vi "DataTranslation_NM1.vi"() -> ()   [LabVIEW 2011]
doc: "This vi will take data with multiple DT boxes for an arbitrary number of channels either differentially or single ended, depending upon how you have wired the boxes up."
uses:
  Controls/DT_Cluster.ctl
  Controls/DT_Mode.ctl
  Controls/Trigger_Mode.ctl
  Globals/Meas_global.vi
  <userlib>/LV-Link3/PolySubVIs/DtOLTimingSetInput.vi
  <userlib>/LV-Link3/PolySubVIs/DtCreateAinChan.vi
  <userlib>/LV-Link3/PolySubVIs/DtCreateCtrRateChan.vi
  <userlib>/LV-Link3/PolySubVIs/DtOLStartNormal.vi
  <userlib>/LV-Link3/PolySubVIs/DtOLReadMultiple2D.vi
  <userlib>/LV-Link3/PolySubVIs/DtOLTriggerDigital.vi
panel:
  out "DAQ Error":errorcluster
  out "Array":T1[](array[typedef])
  out "Clock Task":i32
  out "Waveform Graph":dbl[][](graph)
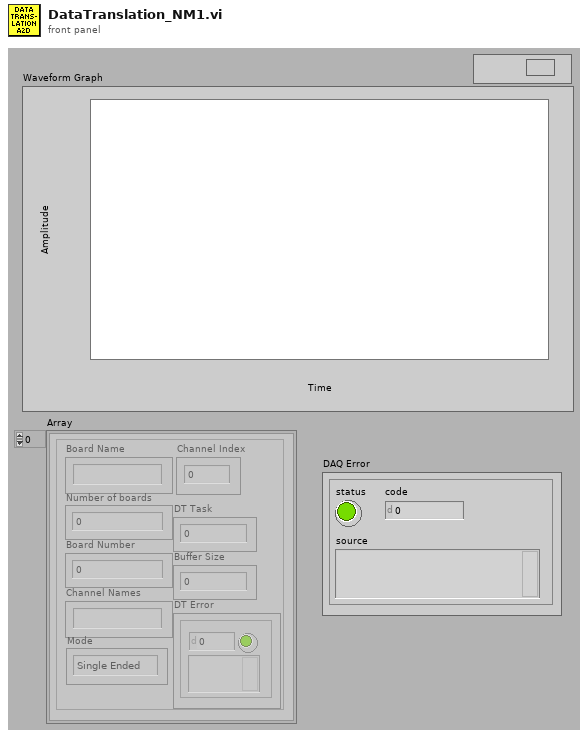
[diagram p1: front panel]
types:
  T1 = typedef "DT_Cluster.ctl" = cluster{"Board Name":string, "Number of boards":u32, "Board Number":u32, "Channel Names":string, "Channel Index":i32[], "DT Task":i32, "DT Error":errorcluster, "Mode":T2, "Buffer Size":u32}
  T2 = typedef "DT_Mode.ctl" = enum16{"Single Ended", "Differential"}
  T3 = typedef "Trigger_Mode.ctl" = enum16{"Free Running", "Start on Trigger", "Trigger Every Block", "Trigger Every Sample"}
  T4 = enum32{"Internal Clock", "External Clock", "No Timing"}
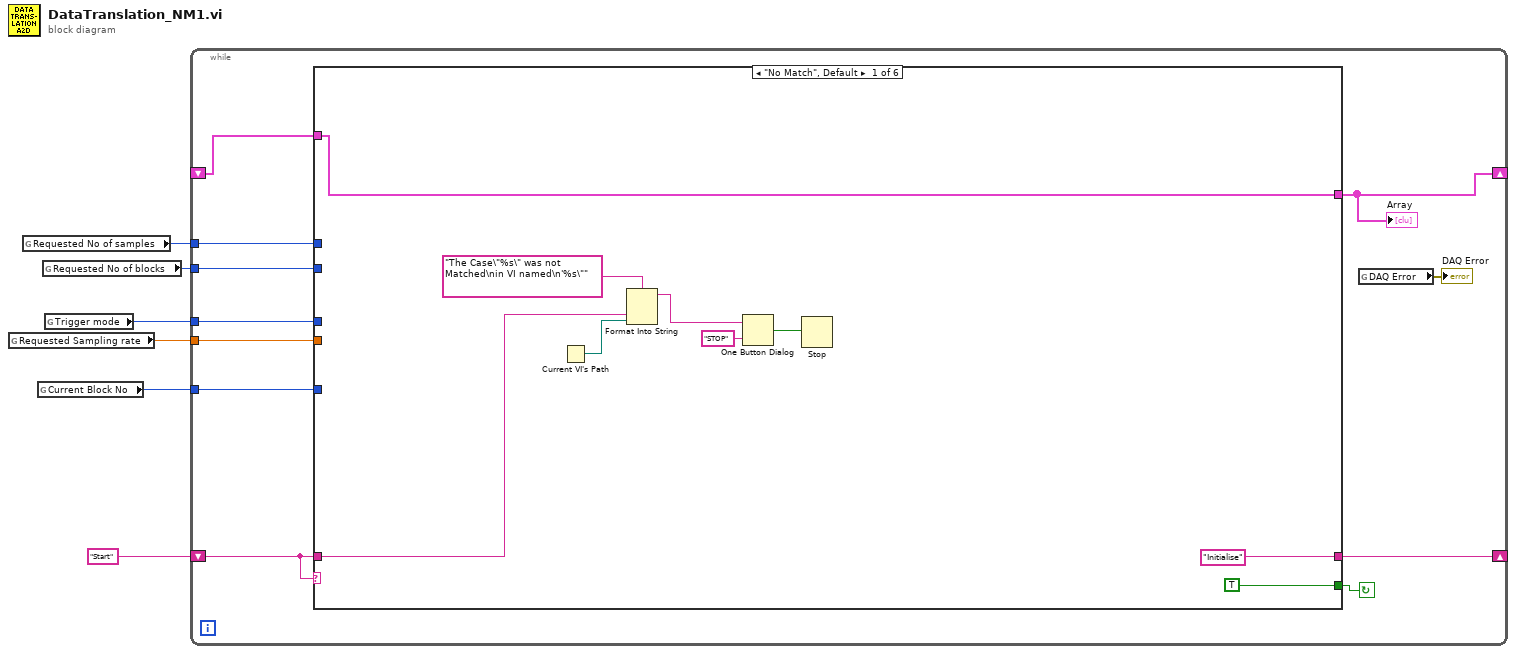
[diagram p0: block diagram]
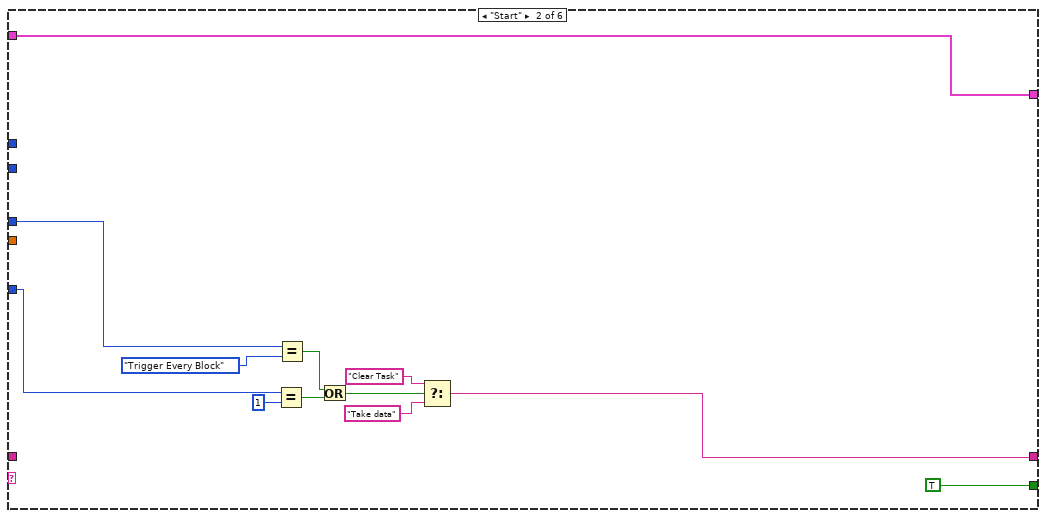
[diagram p2: hidden frame]
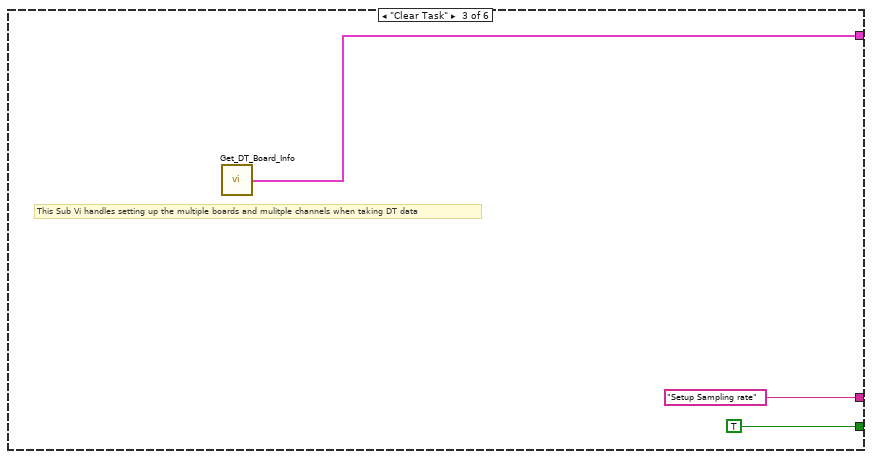
[diagram p3: hidden frame]
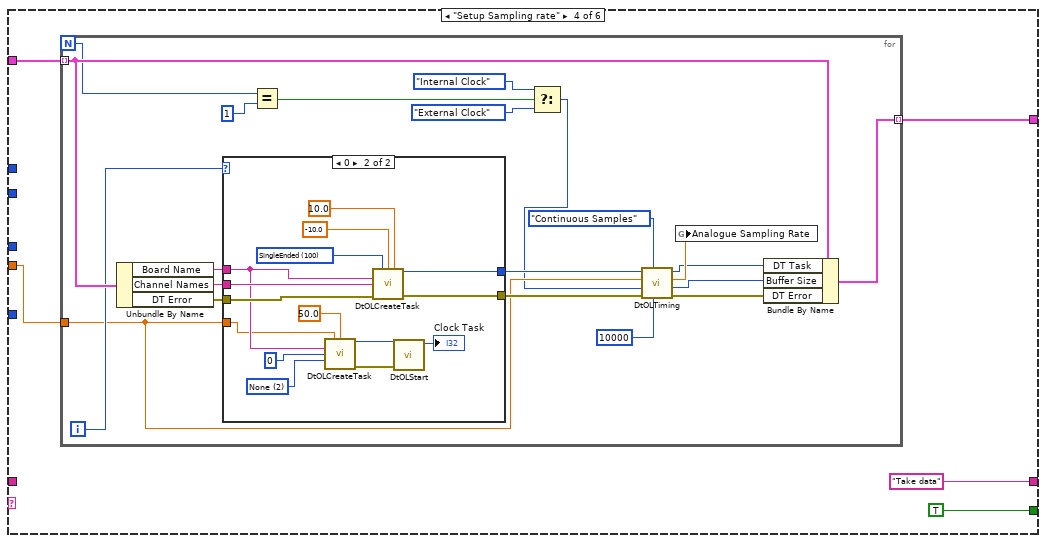
[diagram p4: hidden frame]
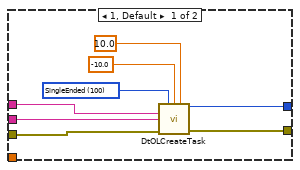
[diagram p5: hidden frame]
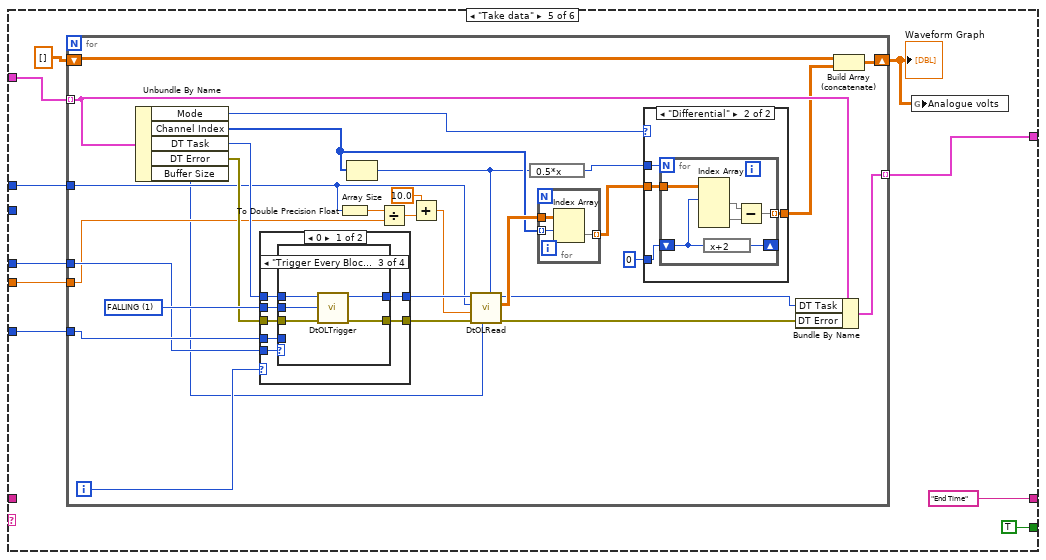
[diagram p6: hidden frame]
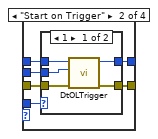
[diagram p9: hidden frame]
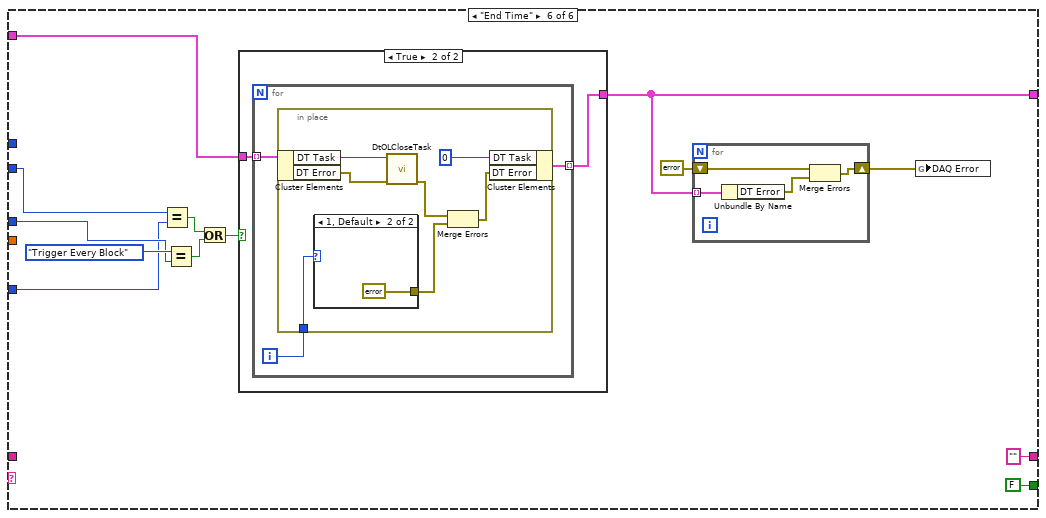
[diagram p13: hidden frame]
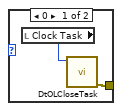
[diagram p15: hidden frame]
diagram:
  n1 = global read "Meas_global.vi" "Requested Sampling rate"() -> (w5:dbl)
  n2 = global read "Meas_global.vi" "Requested No of samples"() -> (w4:i32)
  n3 = global read "Meas_global.vi" "Current Block No"() -> (w2:i32)
  n4 = global read "Meas_global.vi" "Requested No of blocks"() -> (w1:i32)
  n5 = global read "Meas_global.vi" "Trigger mode"() -> (w3:T3)
  n6 = while {
    shift-left: "Start" -> [w16]
    shift-right: [w17] -> _
    tunnel: w5 -> [w15]
    tunnel: w4 -> [w14]
    tunnel: w2 -> [w13]
    tunnel: w3 -> [w11]
    tunnel: w1 -> [w10]
    shift-right: [w9] -> _
    shift-left: _ -> [w8]
    stop <- w12 continue-if-true
    n7 = case shown="\"No Match\", Default" w16 {
      tunnel: ["Initialise" w38 "Setup Sampling rate" "Take data" "End Time" "" ("f")] -> w17
      tunnel: w16 -> [w22 _ _ _ _ _]
      tunnel: w15 -> [_ _ _ w46 w92 _]
      tunnel: w14 -> [_ _ _ _ w99 _]
      tunnel: w13 -> [_ w34 _ _ w97 w180]
      tunnel: [TRUE TRUE TRUE TRUE TRUE FALSE] -> w12
      tunnel: w11 -> [_ w32 _ _ w96 w181]
      tunnel: w10 -> [_ _ _ _ _ w182]
      tunnel: w8 -> [w18 w27 _ w43 w95 w178]
      tunnel: [w18 w27 w39 w42 w94 w177] -> w9
      frame "No Match", Default {
        (unwired) FALSE
        n8 = Current VI's Path() -> (path=w21:path)
        n9 = Format Into String(format string="The Case\"%s\" was not Matched\nin VI named\n'%s\"" ("Format String"), w22, w21) -> (resulting string=w25:string)  [unwired: 2 in, 1 out]
        n10 = One Button Dialog(message=w25, button name ("OK")="STOP") -> (true=w23:bool)
        n11 = Stop(stop? (T)=w23) -> ()
      }
      frame "Start" {
        (unwired) TRUE
        n12 = Equal?(x=w34, y=1) -> (x = y?=w30:bool)
        n13 = Equal?(x=w32, y=Trigger_Mode."Trigger Every Block") -> (x = y?=w29:bool)
        n14 = Or(x=w29, y=w30) -> (x .or. y?=w28:bool)
        n15 = Select(t="Clear Task", s=w28, f="Take data") -> (s? t:f=w38:string)
      }
      frame "Clear Task" {
        (unwired) TRUE
        # "This Sub Vi handles setting up the multiple boards and mulitple channels when taking DT data"
        n16 = call "Get_DT_Board_Info.vi"() -> ("DT Cluster Array"=w39:T1[])  [unwired: 5 in]
      }
      frame "Setup Sampling rate" {
        n17 = for {
          N -> [w52]
          tunnel: w46 -> [w53]
          tunnel: w43 -> [w60] mode=indexing
          tunnel: [w59] -> w42 mode=indexing
          i -> [w54]
          n18 = Unbundle By Name(w60) -> ("Board Name"=w63:string, "Channel Names"=w62:string, "DT Error"=w61:errorcluster)
          n19 = case shown="0" w54 {
            tunnel: [w75 w90] -> w66
            tunnel: [w74 w89] -> w65
            tunnel: w63 -> [w73 w83]
            tunnel: w62 -> [w72 w88]
            tunnel: w61 -> [w71 w87]
            tunnel: w53 -> [_ w76]
            frame 1, Default {
              w68 = 100 items=["SingleEnded"=100, "Differential"=101] ("Channel Type")
              n20 = call-poly <userlib>:"DtOLCreateTask.vi"("Channel Type"=w68, "Range Min"=-10.0, "Range Max"=10.0, "Board Name"=w73, "Channel"=w72, "error in (no error)"=w71) -> ("Task out"=w74:i32, "error out"=w75:errorcluster)  [unwired: 7 in, 1 out]
            }
            frame 0 {
              w81 = 2 items=["LowLevel", "HighLevel", "None"] ("Gate Type")
              w84 = 100 items=["SingleEnded"=100, "Differential"=101] ("Channel Type")
              n21 = call-poly <userlib>:"DtOLCreateTask.vi"("Requested\nFrequency (Hz)"=w76, "Duty Cycle"=50.0, "Board Name"=w83, "Counter Num"=u32 0, "Gate Type"=w81) -> ("Task out"=w78:i32, "error out"=w79:errorcluster)  [unwired: 8 in, 1 out]
              n22 = call-poly <userlib>:"DtOLCreateTask.vi"("Channel Type"=w84, "Range Min"=-10.0, "Range Max"=10.0, "Board Name"=w83, "Channel"=w88, "error in (no error)"=w87) -> ("Task out"=w89:i32, "error out"=w90:errorcluster)  [unwired: 7 in, 1 out]
              n23 = call-poly <userlib>:"DtOLStart.vi"("error in (no error)"=w79, "Task in"=w78) -> ("Task out"=→"Clock Task":i32)  [unwired: 8 in, 1 out]
            }
          }
          n24 = Equal?(x=w52, y=1) -> (x = y?=w48:bool)
          n25 = Select(t=T4."Internal Clock" ("Timing"), s=w48, f=T4."External Clock" ("Timing")) -> (s? t:f=w47:T4)
          n26 = call-poly <userlib>:"DtOLTiming.vi"("Num Buffers"=u32 10000, "Sample Mode"=enum16{"Finite Samples", "Continuous Samples"}."Continuous Samples", "error in (no error)"=w66, "Timing"=w47, "Sample Freq (Hz)"=w53, "Task in"=w65) -> ("error out"=w55:errorcluster, "Buffer Size"=w56:u32, "Actual Sample Freq"=w58:dbl, "Task out"=w57:i32)  [unwired: 2 in]
          n27 = global write "Meas_global.vi" "Analogue Sampling Rate"(w58) -> ()
          n28 = Bundle By Name(cluster=w60, "DT Task"=w57, "Buffer Size"=w56, "DT Error"=w55) -> (w59:T1)
        }
      }
      frame "Take data" {
        n29 = for {
          tunnel: w99 -> [w112]
          tunnel: w97 -> [w127]
          tunnel: w96 -> [w126]
          tunnel: w95 -> [w122] mode=indexing
          tunnel: [w121] -> w94 mode=indexing
          shift-right: [w118] -> w91
          shift-left: dbl[][] [] -> [w117]
          tunnel: w92 -> [w113]
          i -> [w110]
          w128 = 1 items=["RISING", "FALLING"] ("External Trigger Polarity")
          n30 = Unbundle By Name(w122) -> ("Mode"=w106:T2, "Channel Index"=w119:i32[], "DT Task"=w125:i32, "DT Error"=w124:errorcluster, "Buffer Size"=w102:u32)
          n31 = case shown="0" w110 {
            tunnel: [w147 w171] -> w129
            tunnel: w128 -> [w146 _]
            tunnel: w127 -> [w145 _]
            tunnel: w126 -> [w144 _]
            tunnel: w125 -> [w143 w171]
            tunnel: w124 -> [w142 w170]
            tunnel: [w141 w170] -> w123
            frame 0 {
              n32 = case shown="\"Trigger Every Block\"" w144 {
                tunnel: [w149 w153 w165 w169] -> w147
                tunnel: w143 -> [w149 w154 w167 w169]
                tunnel: w145 -> [_ w155 _ _]
                tunnel: w146 -> [_ w152 w166 _]
                tunnel: w142 -> [w148 w151 w164 w168]
                tunnel: [w148 w150 w163 w168] -> w141
                frame "Free Running" {
                }
                frame "Start on Trigger" {
                  n33 = case shown="1" w155 {
                    tunnel: w154 -> [w160 w162]
                    tunnel: w151 -> [w159 w161]
                    tunnel: [w157 w162] -> w153
                    tunnel: [w158 w161] -> w150
                    tunnel: w152 -> [w156 _]
                    frame 1 {
                      n34 = call-poly <userlib>:"DtOLTrigger.vi"("error in (no error)"=w159, "External Trigger Polarity"=w156, "Task in"=w160) -> ("error out"=w158:errorcluster, "Task out"=w157:i32)  [unwired: 7 in]
                    }
                    frame 2, Default {
                    }
                  }
                }
                frame "Trigger Every Block" {
                  n35 = call-poly <userlib>:"DtOLTrigger.vi"("error in (no error)"=w164, "External Trigger Polarity"=w166, "Task in"=w167) -> ("error out"=w163:errorcluster, "Task out"=w165:i32)  [unwired: 7 in]
                }
                frame "Trigger Every Sample" {
                }
              }
            }
            frame 1, Default {
            }
          }
          n36 = To Double Precision Float(number=w112) -> (double precision float=w116:dbl)
          n37 = Array Size(array=w119) -> (size(s)=w104:i32)
          n38 = Divide(x=w116, y=w113) -> (x/y=w115:dbl)
          n39 = Add(x=10.0, y=w115) -> (x+y=w111:dbl)
          n40 = call-poly <userlib>:"DtOLRead.vi"("Number Chan to Read"=w104, "Buffer size"=w102, "error in (no error)"=w123, "Timeout"=w111, "Samples Per Channel"=w112, "Task in"=w129) -> ("error out"=w101:errorcluster, "2D Data out"=w120:dbl[][], "Task out"=w109:i32)  [unwired: 1 in, 2 out]
          n41 = expression code="0.5*x"(w104) -> (w103:i32)
          n42 = for {
            tunnel: w119 -> [w174] mode=indexing
            tunnel: w120 -> [w173]
            tunnel: [w172] -> w108 mode=indexing
            n43 = Index Array(array=w173, index (row)=w174) -> (element=w172:dbl[])  [unwired: 1 in]
          }
          n44 = case shown="\"Differential\"" w106 {
            tunnel: w108 -> [w130 w134]
            tunnel: [w130 w133] -> w107
            tunnel: 0 ("size(s)") -> [_ w132]
            tunnel: w103 -> [_ w131]
            frame "Single Ended", Default {
            }
            frame "Differential" {
              n45 = for {
                N: w131 -> [_]
                tunnel: w134 -> [w140]
                shift-right: [w139] -> _
                shift-left: w132 -> [w138]
                tunnel: [w136] -> w133 mode=indexing
                n46 = Index Array(array=w140, index (row) #1=w138) -> (element #1=w135:dbl[], element #2=w137:dbl[])  [unwired: 3 in]
                n47 = expression code="x+2"(w138) -> (w139:i32)
                n48 = Subtract(x=w135, y=w137) -> (x-y=w136:dbl[])
              }
            }
          }
          n49 = Bundle By Name(cluster=w122, "DT Task"=w109, "DT Error"=w101) -> (w121:T1)
          n50 = Build Array (concatenate)(w117, w107) -> (w118:dbl[][])
        }
        "Waveform Graph" <- w91
        n51 = global write "Meas_global.vi" "Analogue volts"(w91) -> ()
      }
      frame "End Time" {
        n52 = Equal?(x=w182, y=w180) -> (x = y?=w184:bool)
        n53 = Equal?(x=Trigger_Mode."Trigger Every Block", y=w181) -> (x = y?=w183:bool)
        n54 = Or(x=w184, y=w183) -> (x .or. y?=w179:bool)
        n55 = case shown="True" w179 {
          tunnel: w178 -> [w192 w194]
          tunnel: [w192 w193] -> w177
          frame False {
          }
          frame True {
            n56 = for {
              tunnel: w194 -> [w197] mode=indexing
              tunnel: [w196] -> w193 mode=indexing
              i -> [w195]
              n57 = in-place {
                in-place-border: w195 -> [w198]
                n58 = in-place-cluster #1(w197) -> ("DT Task"=w204:i32, "DT Error"=w203:errorcluster)
                n59 = case shown="1, Default" w198 {
                  tunnel: [w205 errorcluster {"status"=FALSE, "code"=0, "source"=""} ("Error Out")] -> w202
                  frame 0 {
                    n60 = local read "Clock Task"() -> (w206:i32)
                    n61 = call <userlib>:"DtOLCloseTask.vi"("Task in"=w206) -> ("Error Out"=w205:errorcluster)  [unwired: 10 in]
                  }
                  frame 1, Default {
                  }
                }
                n62 = call <userlib>:"DtOLCloseTask.vi"("Error in"=w203, "Task in"=w204) -> ("Error Out"=w201:errorcluster)  [unwired: 9 in]
                n63 = Merge Errors(w201, w202) -> (w200:errorcluster)
                n64 = in-place-cluster #1("DT Task"=0, "DT Error"=w200) -> (w196:T1)
              }
            }
          }
        }
        n65 = for {
          tunnel: w177 -> [w191] mode=indexing
          shift-right: [w188] -> w175
          shift-left: errorcluster {"status"=FALSE, "code"=0, "source"=""} ("error IO") -> [w189]
          n66 = Unbundle By Name(w191) -> ("DT Error"=w190:errorcluster)
          n67 = Merge Errors(w189, w190) -> (w188:errorcluster)
        }
        n68 = global write "Meas_global.vi" "DAQ Error"(w175) -> ()
      }
    }
    "Array" <- w9
    n69 = global read "Meas_global.vi" "DAQ Error"() -> (→"DAQ Error":errorcluster)
  }
